vi "Caller.vi"(6 "Sub Panel":refnum<vi>, 8 "Error In":errorcluster, 10 "Data Value Reference In":refnum<data-value>, 11 "NumericOperation in":refnum<class "NumericOperation.lvclass">) -> (0 "Error Out":errorcluster, 3 "NumericOperation out":refnum<class "NumericOperation.lvclass">)   [LabVIEW 2021, in "Calculator.lvlib" / "NumericOperation.lvclass"]
doc: "This VI is an overriding method which overrides to its child classes based on the object wired which asynchronously calls the UI.vi to be opened in subpanel."
uses:
  NumericOperation.lvclass
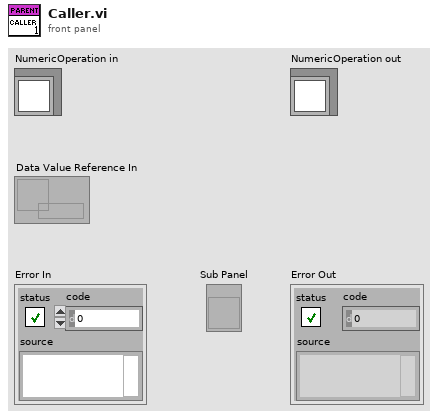
[diagram p1: front panel]
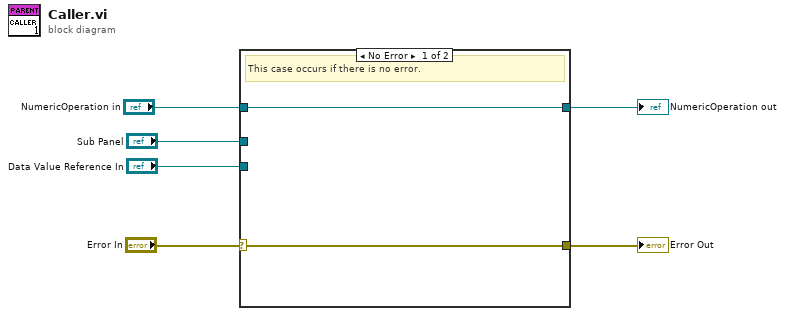
[diagram p0: block diagram]
diagram:
  n1 = case shown="No Error" "Error In" {
    selector: "Error In" -> [w7 w10]
    tunnel: [w7 w10] -> w5
    tunnel: [w8 w9] -> w3
    tunnel: "NumericOperation in" -> [w8 w9]
    tunnel: "Sub Panel" -> [_ _]
    tunnel: "Data Value Reference In" -> [_ _]
    frame No Error {
      # "This case occurs if there is no error."
    }
    frame Error {
      # "This case occurs if there is any error."
    }
  }
  "Error Out" <- w5
  "NumericOperation out" <- w3
